vi "Com _Send Email.vi"(0 "Traceability 引用句柄":refnum<k24>, 1 "sSubject":string, 2 "sUserNo":string, 5 "sTo":string, 7 "sCC":string, 9 "sFrom":string, 11 "error in (no error)":errorcluster caption="错误输入（无错误）", 12 "sComment":string) -> (4 "Traceability 引用句柄输出":refnum<k24>, 6 "Com_SendEmail":string, 15 "error out":errorcluster caption="错误输出")   [LabVIEW 2014, in "Traceability.lvlib"]
uses:
  D:/webservice/Traceability.dll
  Traceability.dll
  Traceability.lvlib
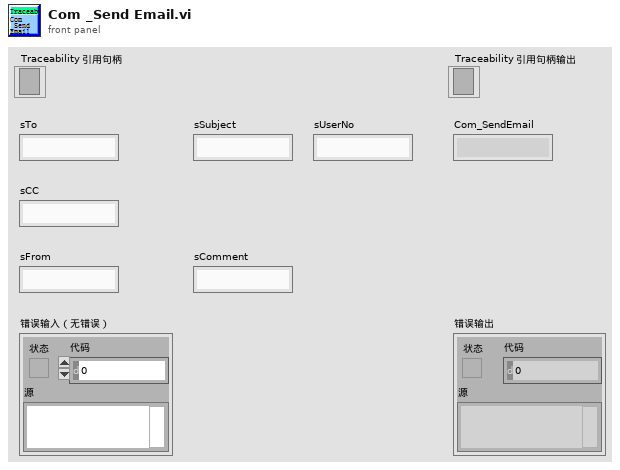
[diagram p1: front panel]
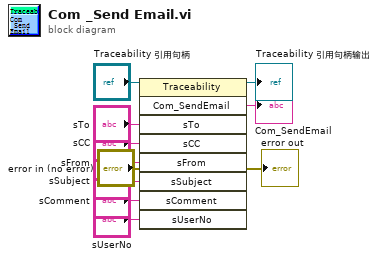
[diagram p0: block diagram]
diagram:
  n1 = invoke class="Traceability" method="Com_SendEmail"(reference="Traceability 引用句柄", error in="error in (no error)", "sTo"="sTo", "sCC"="sCC", "sFrom"="sFrom", "sSubject"="sSubject", "sComment"="sComment", "sUserNo"="sUserNo") -> (reference out=→"Traceability 引用句柄输出":refnum<k24>, error out=→"error out":errorcluster, "Com_SendEmail"=→"Com_SendEmail":string)  [unwired: 1 in, 6 out]
